vi "Main.vi"() -> ()   [LabVIEW 2018]
uses:
  <vilib>/httpClient/LabVIEWHTTPClient.lvlib
panel:
  out "No of Car Manufacturers Remaining":i32
  out "No of Cars Remaining":i32
  out "All Car Dimensions":string[][](array[string])
  out "Dimensions Fetched":string[][](array[string])
  out "Model HTMLs":string[](array[string])
  out "No of HTMLs":i32
  out "Car HTMLs":string[](array[string])
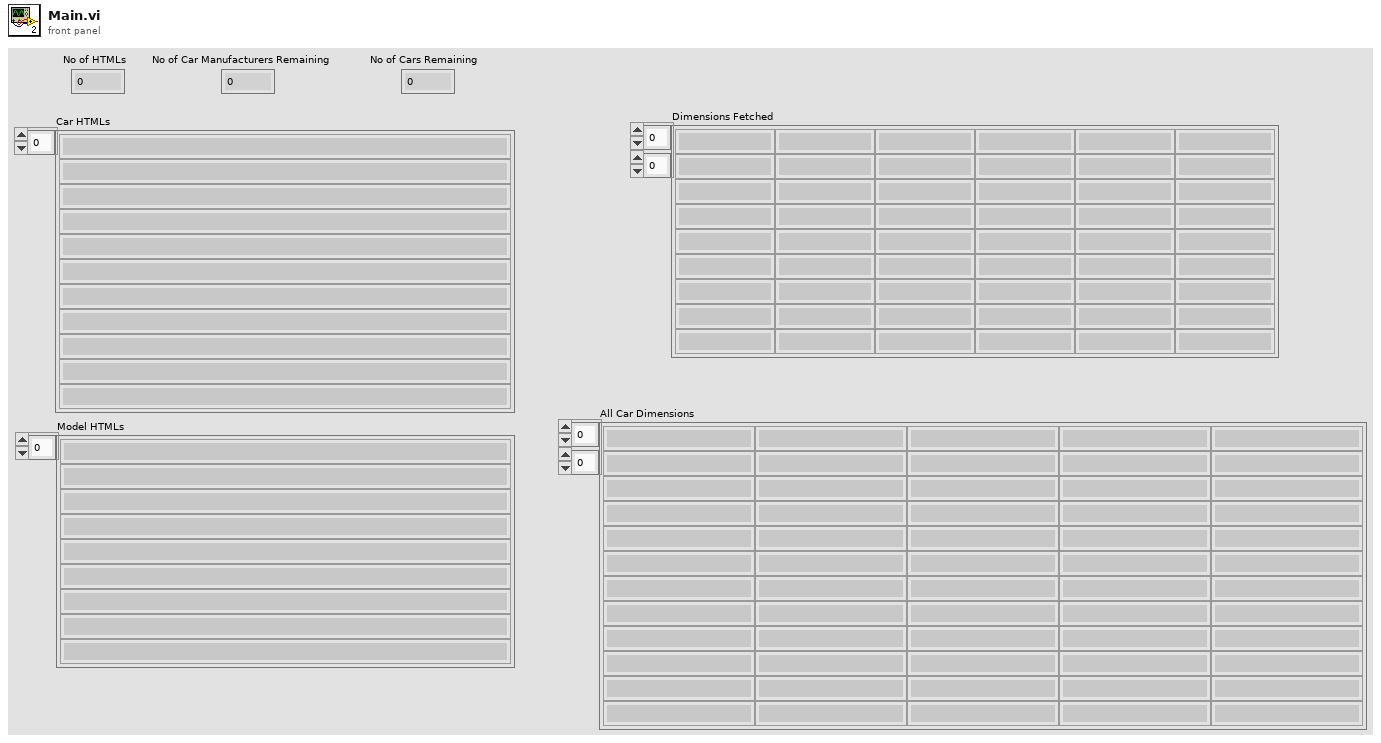
[diagram p1: front panel]
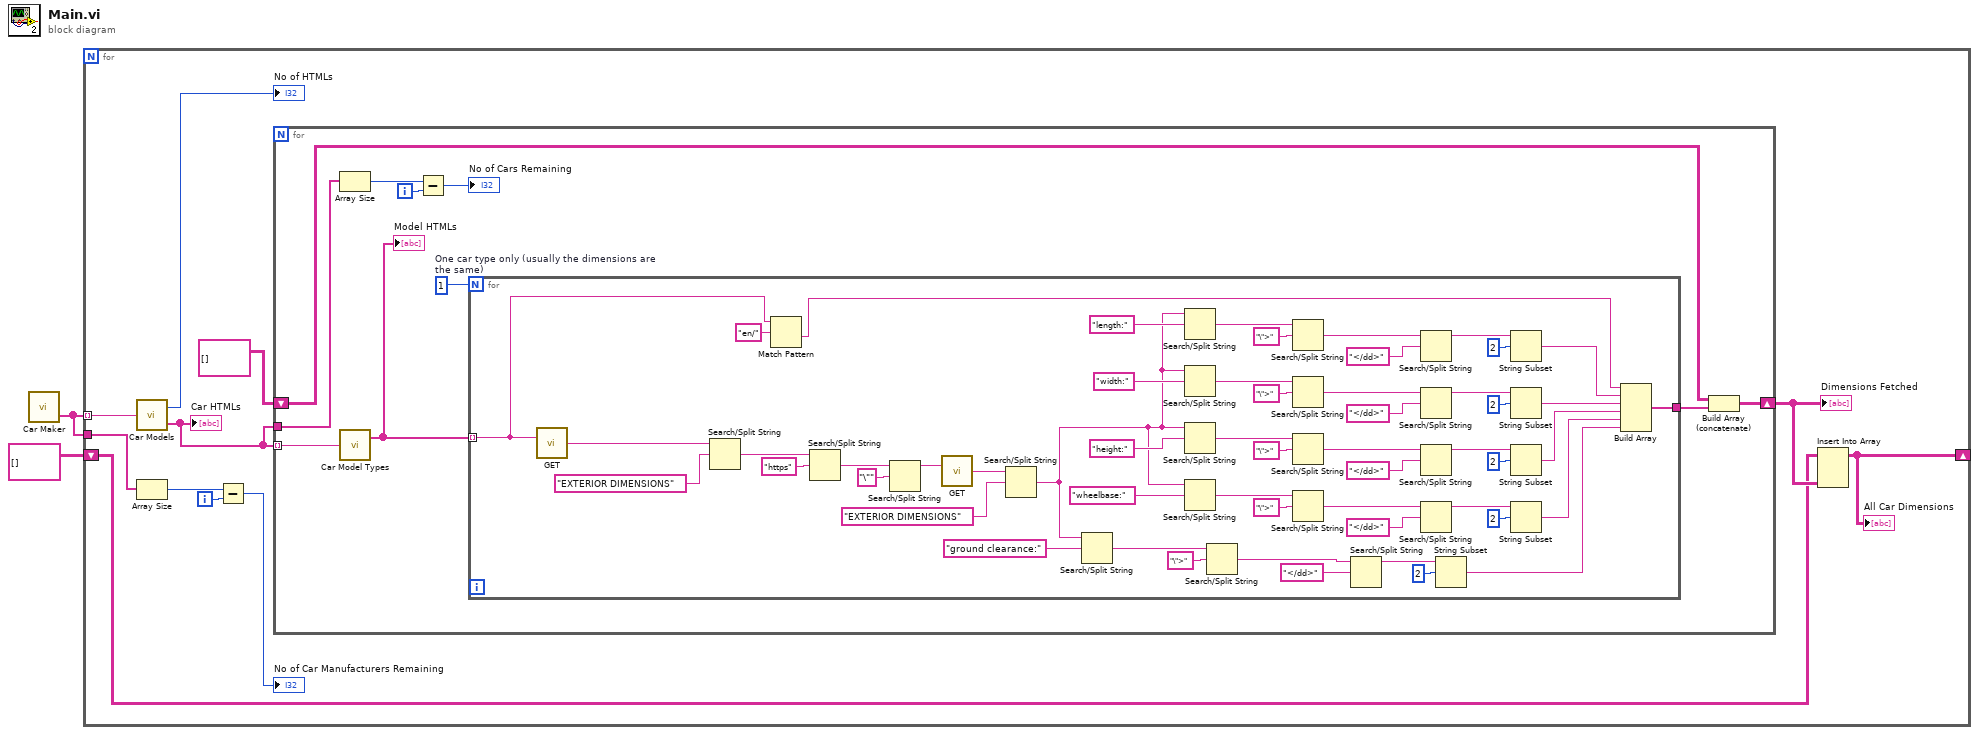
[diagram p0: block diagram]
diagram:
  n1 = call "Car Maker.vi"() -> ("HTMLs"=w1:string[])  [unwired: 1 out]
  n2 = for {
    tunnel: w1 -> [w13] mode=indexing
    shift-right: [w3] -> _
    shift-left: string[][] [] -> [w9]
    tunnel: w1 -> [w7]
    i -> [w6]
    n3 = call "Car Models.vi"("body"=w13) -> ("No of HTMLs"=→"No of HTMLs":i32, "Car HTMLs"=w8:string[])
    "Car HTMLs" <- w8
    n4 = Array Size(array=w7) -> (size(s)=w5:i32)
    n5 = Subtract(x=w5, y=w6) -> (x-y=→"No of Car Manufacturers Remaining":i32)
    n6 = for {
      tunnel: w8 -> [w22] mode=indexing
      shift-right: [w19] -> w10
      shift-left: string[][] [] -> [w18]
      tunnel: w8 -> [w17]
      i -> [w15]
      w21 = 1  # One car type only (usually the dimensions are the same)
      n7 = Array Size(array=w17) -> (size(s)=w16:i32)
      n8 = call "Car Model Types.vi"("body"=w22) -> ("Car HTMLs"=w23:string[])  [unwired: 1 out]
      "Model HTMLs" <- w23
      n9 = Subtract(x=w16, y=w15) -> (x-y=→"No of Cars Remaining":i32)
      n10 = for {
        N: w21 -> [_]
        tunnel: w23 -> [w26] mode=indexing
        tunnel: [w27] -> w20
        n11 = call <vilib>:"GET.vi"("url"=w26) -> ("body"=w77:string)  [unwired: 11 in, 3 out]
        n12 = Search/Split String(string=w77, search string/char (-)="EXTERIOR DIMENSIONS" ("string")) -> (match + rest of string=w72:string)  [unwired: 1 in, 2 out]
        n13 = Match Pattern(string=w26, regular expression="en/") -> (after substring=w24:string)  [unwired: 1 in, 3 out]
        n14 = Search/Split String(string=w72, search string/char (-)="https") -> (match + rest of string=w74:string)  [unwired: 1 in, 2 out]
        n15 = Search/Split String(string=w74, search string/char (-)="\"") -> (substring before match=w62:string)  [unwired: 1 in, 2 out]
        n16 = call <vilib>:"GET.vi"("url"=w62) -> ("body"=w63:string)  [unwired: 11 in, 3 out]
        n17 = Search/Split String(string=w63, search string/char (-)="EXTERIOR DIMENSIONS" ("string")) -> (match + rest of string=w33:string)  [unwired: 1 in, 2 out]
        n18 = Search/Split String(string=w33, search string/char (-)="ground clearance:") -> (match + rest of string=w38:string)  [unwired: 1 in, 2 out]
        n19 = Search/Split String(string=w33, search string/char (-)="length:") -> (match + rest of string=w68:string)  [unwired: 1 in, 2 out]
        n20 = Search/Split String(string=w33, search string/char (-)="width:") -> (match + rest of string=w57:string)  [unwired: 1 in, 2 out]
        n21 = Search/Split String(string=w33, search string/char (-)="height:") -> (match + rest of string=w52:string)  [unwired: 1 in, 2 out]
        n22 = Search/Split String(string=w33, search string/char (-)="wheelbase:") -> (match + rest of string=w43:string)  [unwired: 1 in, 2 out]
        n23 = Search/Split String(string=w38, search string/char (-)="\">") -> (match + rest of string=w36:string)  [unwired: 1 in, 2 out]
        n24 = Search/Split String(string=w68, search string/char (-)="\">") -> (match + rest of string=w66:string)  [unwired: 1 in, 2 out]
        n25 = Search/Split String(string=w57, search string/char (-)="\">") -> (match + rest of string=w59:string)  [unwired: 1 in, 2 out]
        n26 = Search/Split String(string=w52, search string/char (-)="\">") -> (match + rest of string=w50:string)  [unwired: 1 in, 2 out]
        n27 = Search/Split String(string=w43, search string/char (-)="\">") -> (match + rest of string=w45:string)  [unwired: 1 in, 2 out]
        n28 = Search/Split String(string=w36, search string/char (-)="</dd>") -> (substring before match=w35:string)  [unwired: 1 in, 2 out]
        n29 = Search/Split String(string=w66, search string/char (-)="</dd>") -> (substring before match=w65:string)  [unwired: 1 in, 2 out]
        n30 = Search/Split String(string=w59, search string/char (-)="</dd>") -> (substring before match=w60:string)  [unwired: 1 in, 2 out]
        n31 = Search/Split String(string=w50, search string/char (-)="</dd>") -> (substring before match=w49:string)  [unwired: 1 in, 2 out]
        n32 = Search/Split String(string=w45, search string/char (-)="</dd>") -> (substring before match=w46:string)  [unwired: 1 in, 2 out]
        n33 = String Subset(string=w35, offset (0)=2) -> (substring=w28:string)  [unwired: 1 in]
        n34 = String Subset(string=w65, offset (0)=2) -> (substring=w32:string)  [unwired: 1 in]
        n35 = String Subset(string=w60, offset (0)=2) -> (substring=w31:string)  [unwired: 1 in]
        n36 = String Subset(string=w49, offset (0)=2) -> (substring=w30:string)  [unwired: 1 in]
        n37 = String Subset(string=w46, offset (0)=2) -> (substring=w29:string)  [unwired: 1 in]
        n38 = Build Array(w24, w32, w31, w30, w29, w28) -> (w27:string[])
      }
      n39 = Build Array (concatenate)(w18, w20) -> (w19:string[][])
    }
    "Dimensions Fetched" <- w10
    n40 = Insert Into Array(array=w9, new element=w10) -> (w3:string[][])  [unwired: 2 in]
    "All Car Dimensions" <- w3
  }
